vi "Sort Parent Infor for Children.vi"(8 "Error In":errorcluster, 10 "Additional Labels":string[][](array[string]), 11 "Control Information in":string[][](array[string])) -> (0 "Error Out":errorcluster, 2 "Control Names":string[](array[string]), 3 "Broken Out Additional Labels":string[][][](array[string]))   [LabVIEW 2017, in "Localization.lvlib"]
doc: "TAkes the Control Items and Additional Information and sorts the additional information to be added to sub elements. Of a cluster is separates the information of the cluster into the information that gets written into the specific controls of the cluster.\n\nChoose Movement Consulting, LLC"
uses:
  Localization.lvlib
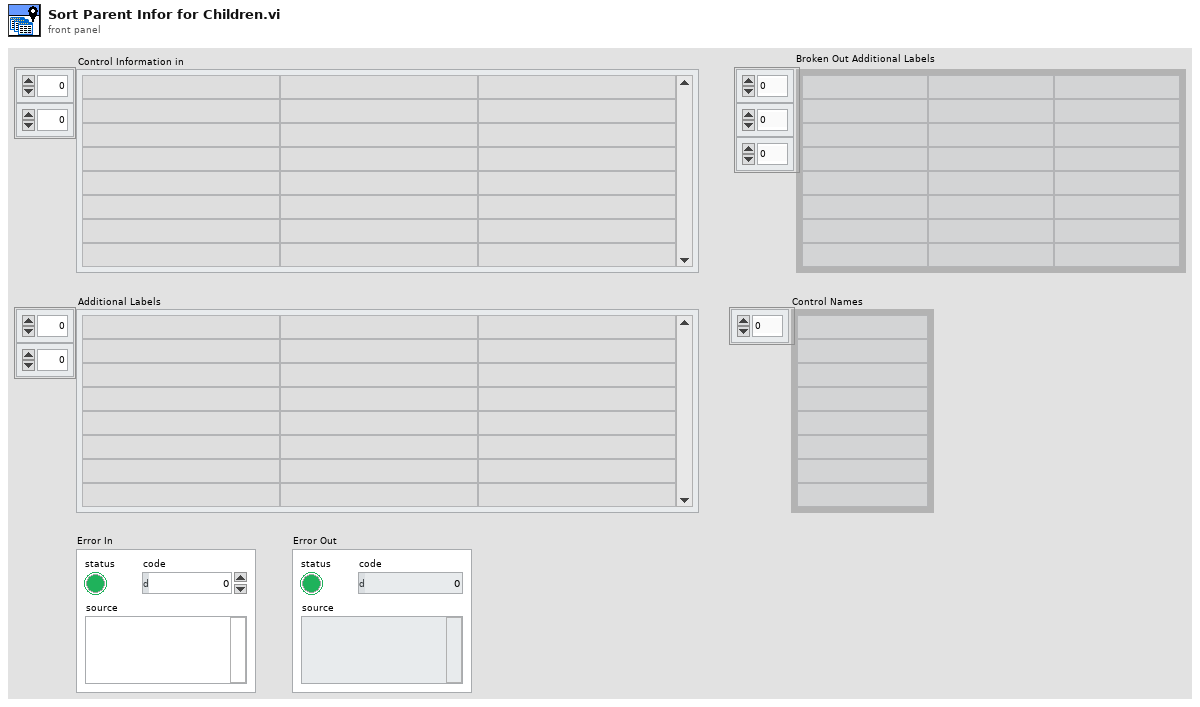
[diagram p1: front panel]
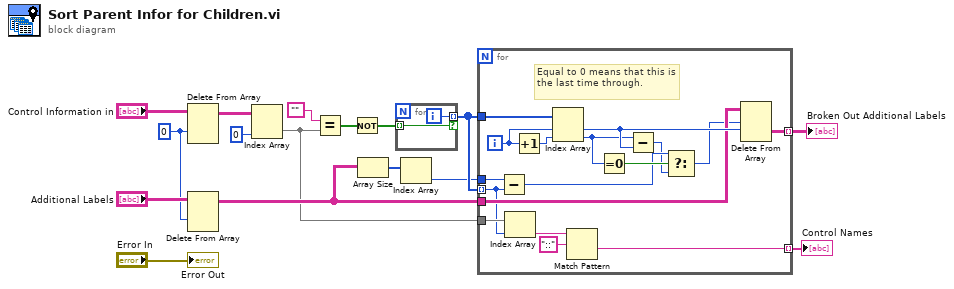
[diagram p0: block diagram]
diagram:
  w14 = 0 ("index (row)")
  n1 = Delete From Array(array="Control Information in", index (row)=w14) -> (array with subset deleted=w9:string[][])  [unwired: 2 in, 1 out]
  n2 = Delete From Array(array="Additional Labels", index (row)=w14) -> (array with subset deleted=w5:string[][])  [unwired: 2 in, 1 out]
  n3 = Index Array(array=w9, index (col)=0 ("disabled index (col)")) -> (element=w2:string[])  [unwired: 1 in]
  n4 = Equal?(x="", y=w2) -> (x = y?=w10:bool[])
  n5 = Not(x=w10) -> (.not. x?=w7:bool[])
  n6 = Array Size(array=w5) -> (size(s)=w4:i32[])
  n7 = for {
    tunnel: w7 -> [w17] mode=indexing
    tunnel: [w18] -> w6 mode=indexing if=w17
    i -> [w18]
  }
  n8 = Index Array(array=w4) -> (element=w3:i32)  [unwired: 1 in]
  n9 = for {
    tunnel: w6 -> [w35]
    tunnel: [w31] -> w8 mode=indexing
    tunnel: w6 -> [w22] mode=indexing
    tunnel: w5 -> [w30]
    tunnel: w3 -> [w27]
    tunnel: w2 -> [w23]
    tunnel: [w19] -> w1 mode=indexing
    i -> [w34]
    # "Equal to 0 means that this is the last time through."
    n10 = Subtract(x=w27, y=w22) -> (x-y=w26:i32)
    n11 = Index Array(array=w23, index=w22) -> (element=w21:string)
    n12 = Increment(x=w34) -> (x+1=w33:i32)
    n13 = Index Array(array=w35, index #1=w34, index #2=w33) -> (element #1=w32:i32, element #2=w29:i32)
    n14 = Match Pattern(string=w21, regular expression="::") -> (after substring=w19:string)  [unwired: 1 in, 3 out]
    n15 = Equal To 0?(x=w29) -> (x = 0?=w28:bool)
    n16 = Subtract(x=w29, y=w32) -> (x-y=w25:i32)
    n17 = Select(t=w26, s=w28, f=w25) -> (s? t:f=w24:i32)
    n18 = Delete From Array(array=w30, length=w24, index (row)=w32) -> (deleted portion=w31:string[][])  [unwired: 1 in, 1 out]
  }
  "Broken Out Additional Labels" <- w8
  "Control Names" <- w1
  "Error Out" <- "Error In"
